vi "Kalibrierung laden.vi"() -> ()   [LabVIEW 2020, in "FT-IR.lvlib" / "Spanfaktor.lvlib"]
uses:
  Spanfaktor.lvlib
  FGV FT-IR Aktionen.ctl
  Sprachverwaltung/FGV Aktion Tabelle zerlegen.ctl
  FGV FT-IR Gasliste Aktionen.ctl
  Aktion FGV Span.ctl
  Aktionen EVID-Codes.ctl
  FT-IR.lvlib
  Allgemein/allgemeine Sub-VIs.lvlib
  TOOLweb Interface Library/TOOLweb Interface.lvlib
  Sprachverwaltung/Sprachverwaltung.lvlib
panel:
  out "Offset alt":string
  out "Offset neu":string
  out "Spanfaktor alt":string
  out "Spanfaktor Neu":string caption="Spanfaktor neu"
  out "Kalibrierung für Komponente":string
  # "Kalibrierdaten laden"
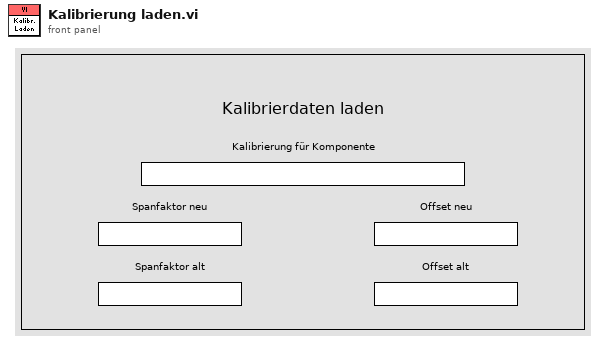
[diagram p1: front panel]
types:
  T1 = typedef "Sprachverwaltung.lvlib/FGV Aktion Tabelle zerlegen.ctl" = enum16{"laden", "vereinzeln", "speichern"}
  T2 = typedef "FT-IR.lvlib/FGV FT-IR Aktionen.ctl" = enum16{"lesen", "NOG setzen", "NOS setzen", "Initialisieren", "speichern", "ALLES setzen", "FT-IR Spektrum loggen", "Komm Stoppen", "Spektrum LogKonfig"}
  T3 = typedef "FT-IR.lvlib/Aktionen EVID-Codes.ctl" = enum16{"lesen", "setzen", "laden", "speichern", "1Hz/5Hz", "Smoothing", "Rolling Average"}
  T4 = typedef "FT-IR.lvlib/FGV FT-IR Gasliste Aktionen.ctl" = enum16{"lesen", "Gasliste FT-IR", "Gasliste ausgelesen", "laden", "speichern", "löschen"}
  T5 = typedef "FT-IR.lvlib/Spanfaktor.lvlib/Aktion FGV Span.ctl" = enum16{"lesen", "Span", "Seite aktiv", "Offset", "FGV aktualisiert", "Aktualisierung aufheben"}
  T6 = typedef "String - Ausgabefeld.ctl" = string
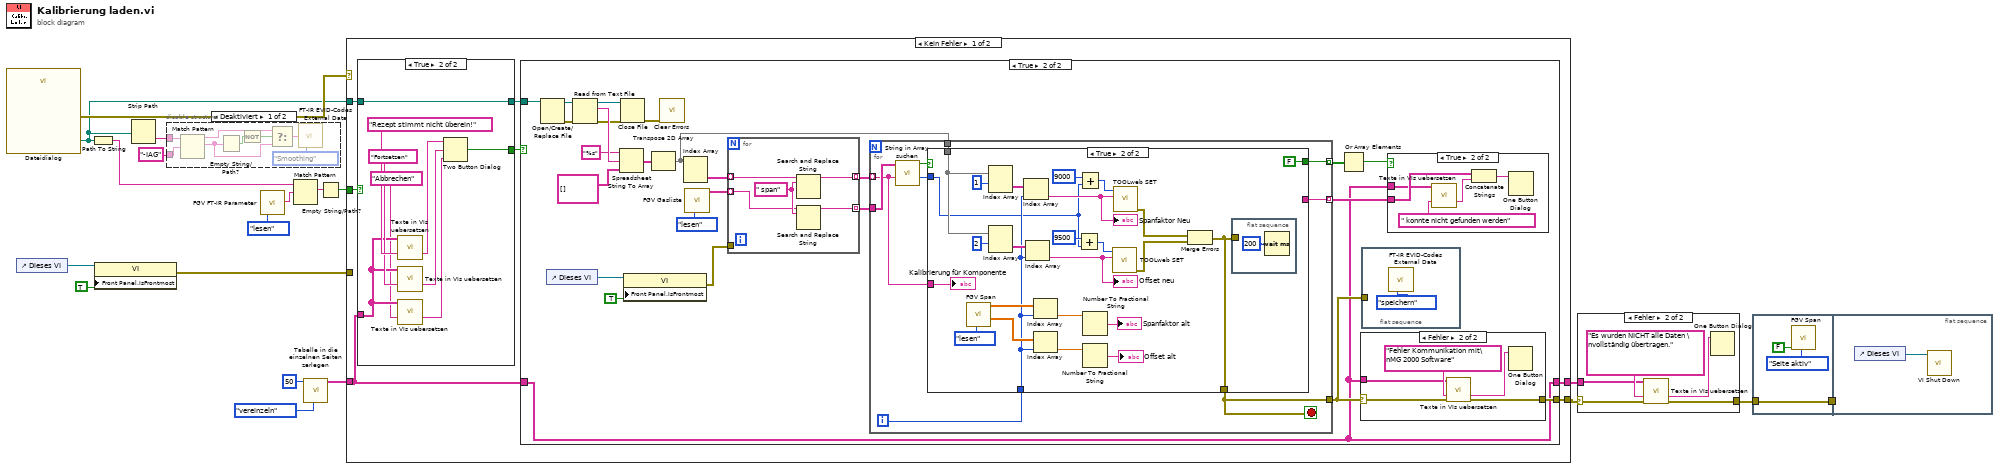
[diagram p0: block diagram]
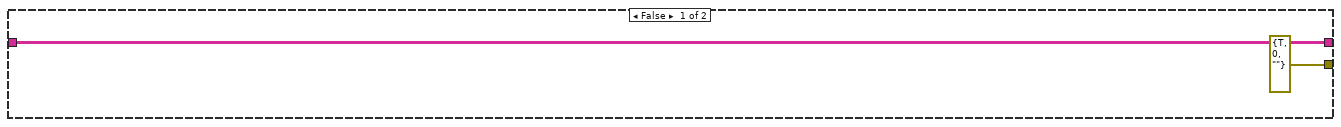
[diagram p3: hidden frame]
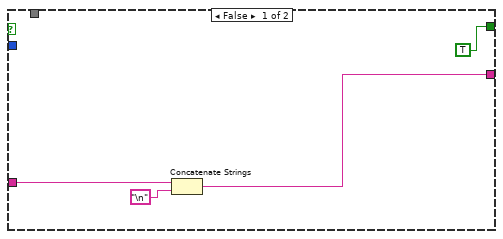
[diagram p6: hidden frame]
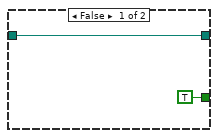
[diagram p7: hidden frame]
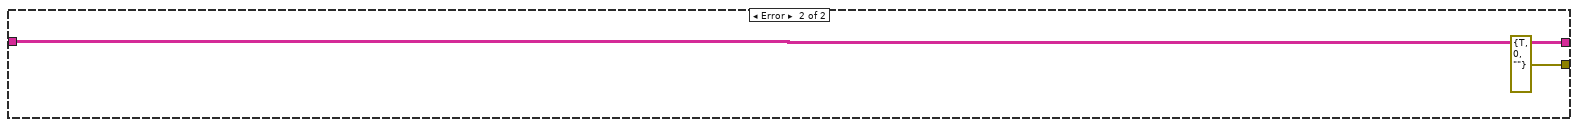
[diagram p8: hidden frame]
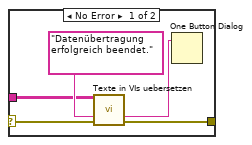
[diagram p9: hidden frame]
diagram:
  n1 = call "Dateidialog"() -> ("selected path"=w9:path, "error out"=w12:errorcluster)  [unwired: 12 in, 2 out]
  n2 = control-ref of="Dieses VI"() -> (w7:refnum<vi>)
  n3 = Path To String(path=w9) -> (string=w10:string)
  n4 = property class="VI"(reference=w7, "Front Panel.IsFrontmost"=TRUE ("Frontpanel-Fenster:Ist im Vordergrund")) -> (error out=w5:errorcluster)  [unwired: 1 in, 1 out]
  n5 = Strip Path(path=w9) -> (name=w8:string)  [unwired: 1 out]
  n6 = disable-structure shown="Deaktiviert" {
    disable-tunnel: "-IAG" ("Regulärer Ausdruck") -> [w27 _]
    disable-tunnel: w8 -> [w25 _]
    frame Disabled {
      n7 = Match Pattern(string=w25, regular expression=w27) -> (before substring=w22:string, match substring=w21:string)  [unwired: 1 in, 2 out]
      n8 = Empty String/Path?(string/path=w21) -> (empty?=w24:bool)
      n9 = Not(x=w24) -> (.not. x?=w20:bool)
      n10 = Select(t=w22, s=w20, f=w21) -> (s? t:f=w23:string)
      n11 = call "FT-IR EVID-Codes External Data.vi"("Rolling Average Settings"=w23, "Aktionen"=Aktionen_EVID-Codes."Smoothing") -> ()  [unwired: 8 in, 6 out]
    }
    frame Enabled {
    }
  }
  n12 = call "FGV FT-IR Parameter.vi"("Aktion"=FGV_FT-IR_Aktionen."lesen") -> ("Current Recipe"=w18:string)  [unwired: 11 in, 7 out]
  n13 = Match Pattern(string=w10, regular expression=w18) -> (match substring=w17:string)  [unwired: 1 in, 3 out]
  n14 = call "Tabelle in die einzelnen Seiten zerlegen.vi"("Aktion"=FGV_Aktion_Tabelle_zerlegen."vereinzeln", "Index (Seite)"=50) -> ("Sprachliste"=w2:string[][])  [unwired: 7 in, 2 out]
  n15 = Empty String/Path?(string/path=w17) -> (empty?=w16:bool)
  n16 = case shown="Kein Fehler" w12 {
    tunnel: w16 -> [w34 _]
    tunnel: w9 -> [w33 _]
    tunnel: [w30 errorcluster {"status"=TRUE, "code"=0, "source"=""} ("error IO")] -> w15
    tunnel: w5 -> [_ _]
    tunnel: w2 -> [w29 w129]
    tunnel: [w28 w129] -> w1
    frame No Error {
      n17 = case shown="True" w34 {
        tunnel: w33 -> [w119 w127]
        tunnel: [TRUE ("T button?") w128] -> w32
        tunnel: [w119 w127] -> w31
        tunnel: w29 -> [_ w122]
        frame False {
        }
        frame True {
          n18 = call "Texte in VIs uebersetzen.vi"("Sprachliste"=w122, "String zum Übersetzen"="Rezept stimmt nicht überein!" ("Nachricht")) -> ("String zum Übersetzen"=w125:string)  [unwired: 9 in, 4 out]
          n19 = call "Texte in VIs uebersetzen.vi"("Sprachliste"=w122, "String zum Übersetzen"="Fortsetzen" ("Text für T-Schaltfläche (\"OK\")")) -> ("String zum Übersetzen"=w123:string)  [unwired: 9 in, 4 out]
          n20 = call "Texte in VIs uebersetzen.vi"("Sprachliste"=w122, "String zum Übersetzen"="Abbrechen" ("Text für F-Schaltfläche (\"Abbrechen\")")) -> ("String zum Übersetzen"=w120:string)  [unwired: 9 in, 4 out]
          n21 = Two Button Dialog(message=w125, 1:w120, 2:w123) -> (T button?=w128:bool)
        }
      }
      n22 = case shown="True" w32 {
        tunnel: w31 -> [_ w52]
        tunnel: [errorcluster {"status"=TRUE, "code"=0, "source"=""} ("error IO") w45] -> w30
        tunnel: w29 -> [w35 w37]
        tunnel: [w35 w37] -> w28
        frame False {
        }
        frame True {
          n23 = Open/Create/Replace File(file path (use dialog)=w52) -> (refnum out=w61:refnum<file>, error out=w53:errorcluster)  [unwired: 1 in, 5 out]
          n24 = control-ref of="Dieses VI"() -> (w39:refnum<vi>)
          n25 = Read from Text File(file (use dialog)=w61, error in=w53) -> (refnum out=w60:refnum<file>, text=w59:string, error out=w56:errorcluster)  [unwired: 3 out]
          n26 = Spreadsheet String To Array(format string="%s" ("Format-String"), spreadsheet string=w59, array type (2D Dbl)=string[][] []) -> (array=w58:string[][])  [unwired: 1 out]
          n27 = Close File(refnum=w60, error in=w56) -> (error out=w57:errorcluster)  [unwired: 1 out]
          n28 = property class="VI"(reference=w39, "Front Panel.IsFrontmost"=TRUE ("Frontpanel-Fenster:Ist im Vordergrund")) -> (error out=w38:errorcluster)  [unwired: 1 in, 1 out]
          n29 = Transpose 2D Array(2D array=w58) -> (transposed array=w46:string[][])
          n30 = call <vilib>:"Clear Errors.vi"("error in (no error)"=w57) -> ()  [unwired: 5 in, 2 out]
          n31 = Index Array(array=w46) -> (element=w50:string[])  [unwired: 2 in]
          n32 = call "FGV Gasliste.vi"("Aktionen"=FGV_FT-IR_Gasliste_Aktionen."lesen") -> ("Aktuelle Gasliste FT-IR"=w49:T6[])  [unwired: 8 in, 2 out]
          n33 = for {
            tunnel: w50 -> [w114] mode=indexing
            tunnel: w49 -> [w113] mode=indexing
            tunnel: [w116] -> w48 mode=indexing
            tunnel: [w115] -> w47 mode=indexing
            tunnel: w38 -> [_]
            w117 = " span"
            n34 = Search and Replace String(input string=w114, search string=w117) -> (result string=w116:string)  [unwired: 6 in, 3 out]
            n35 = Search and Replace String(input string=w113, search string=w117) -> (result string=w115:string)  [unwired: 6 in, 3 out]
          }
          n36 = for {
            tunnel: w48 -> [w78] mode=indexing
            tunnel: w47 -> [w82]
            tunnel: w46 -> [w80]
            tunnel: [w77] -> w44
            tunnel: [w75] -> w41 mode=indexing
            tunnel: [w74] -> w43 mode=indexing
            i -> [w76]
            stop <- w77 stop-if-true
            n37 = call "String in Array suchen.vi"("Nach String/Zeichen suchen (-)"=w78, "String-Array"=w82) -> ("Index"=w79:i32, "Gefunden?"=w81:bool)  [unwired: 7 in, 1 out]
            n38 = case shown="True" w81 {
              tunnel: w80 -> [_ w111]
              tunnel: w79 -> [_ w88]
              tunnel: w78 -> [w86 w108]
              tunnel: [_ w92] -> w77
              tunnel: w76 -> [_ w89]
              tunnel: [w84 _] -> w75
              tunnel: [TRUE FALSE] -> w74
              frame False {
                n39 = Concatenate Strings(w86, "\n") -> (w84:string)
              }
              frame True {
                n40 = call "FGV Span.vi"("Aktion"=Aktion_FGV_Span."lesen") -> ("Offset"=w99:sgl[], "Span"=w100:sgl[])  [unwired: 7 in, 2 out]
                n41 = Index Array(array=w111, index (row)=1 ("Index (Zeile)")) -> (element=w110:string[])  [unwired: 1 in]
                n42 = Index Array(array=w111, index (row)=2 ("Index (Zeile)")) -> (element=w109:string[])  [unwired: 1 in]
                n43 = Index Array(array=w110, index=w89) -> (element=w103:string)
                "Spanfaktor Neu" <- w103
                n44 = Index Array(array=w109, index=w89) -> (element=w102:string)
                "Offset neu" <- w102
                n45 = Index Array(array=w100, index=w89) -> (element=w98:sgl)
                n46 = Index Array(array=w99, index=w89) -> (element=w97:sgl)
                n47 = Add(x=9500, y=w88) -> (x+y=w105:i32)
                n48 = Add(x=9000, y=w88) -> (x+y=w106:i32)
                n49 = Number To Fractional String(number=w98) -> (F-format string=→"Spanfaktor alt":string)  [unwired: 3 in]
                n50 = Number To Fractional String(number=w97) -> (F-format string=→"Offset alt":string)  [unwired: 3 in]
                n51 = call "TOOLweb SET.vi"("Wert-String"=w102, "EVID-Nummer"=w105) -> ("error out"=w93:errorcluster)  [unwired: 3 in, 2 out]
                n52 = call "TOOLweb SET.vi"("Wert-String"=w103, "EVID-Nummer"=w106) -> ("error out"=w94:errorcluster)  [unwired: 3 in, 2 out]
                n53 = Merge Errors(w94, w93) -> (w92:errorcluster)
                n54 = flat-sequence {
                  tunnel: w92 -> [_]
                  frame #0 {
                    n55 = Wait (ms)(milliseconds to wait=u32 200 ("Zu wartende ms")) -> ()  [unwired: 1 out]
                  }
                }
                "Kalibrierung für Komponente" <- w108
              }
            }
          }
          n56 = Or Array Elements(Boolean array=w43) -> (logical OR=w42:bool)
          n57 = case shown="Fehler" w44 {
            selector: w44 -> [w68 w70]
            tunnel: [w68 w69] -> w45
            tunnel: w37 -> [_ w71]
            frame No Error {
            }
            frame Error {
              n58 = call "Texte in VIs uebersetzen.vi"("Sprachliste"=w71, "String zum Übersetzen"="Fehler Kommunikation mit\nMG 2000 Software" ("String"), "error in (no error)"=w70) -> ("String zum Übersetzen"=w73:string, "error out"=w69:errorcluster)  [unwired: 8 in, 3 out]
              n59 = One Button Dialog(message=w73) -> ()  [unwired: 1 in, 1 out]
            }
          }
          n60 = flat-sequence {
            tunnel: w44 -> [_]
            frame #0 {
              n61 = call "FT-IR EVID-Codes External Data.vi"("Aktionen"=Aktionen_EVID-Codes."speichern") -> ()  [unwired: 9 in, 6 out]
            }
          }
          n62 = case shown="True" w42 {
            tunnel: w41 -> [_ w65]
            tunnel: w37 -> [_ w62]
            frame False {
            }
            frame True {
              n63 = call "Texte in VIs uebersetzen.vi"("Sprachliste"=w62, "String zum Übersetzen"=" konnte nicht gefunden werden" ("String")) -> ("String zum Übersetzen"=w63:string)  [unwired: 9 in, 4 out]
              n64 = Concatenate Strings(w65, w63) -> (w66:string)
              n65 = One Button Dialog(message=w66) -> ()  [unwired: 1 in, 1 out]
            }
          }
        }
      }
    }
    frame Error {
    }
  }
  n66 = case shown="Fehler" w15 {
    selector: w15 -> [w134 w138]
    tunnel: [w134 w137] -> w14
    tunnel: w1 -> [w131 w136]
    frame No Error {
      n67 = call "Texte in VIs uebersetzen.vi"("Sprachliste"=w131, "String zum Übersetzen"="Datenübertragung erfolgreich beendet." ("String")) -> ("String zum Übersetzen"=w132:string)  [unwired: 9 in, 4 out]
      n68 = One Button Dialog(message=w132) -> ()  [unwired: 1 in, 1 out]
    }
    frame Error {
      n69 = call "Texte in VIs uebersetzen.vi"("Sprachliste"=w136, "String zum Übersetzen"="Es wurden NICHT alle Daten \nvollständig übertragen." ("String"), "error in (no error)"=w138) -> ("String zum Übersetzen"=w135:string, "error out"=w137:errorcluster)  [unwired: 8 in, 3 out]
      n70 = One Button Dialog(message=w135) -> ()  [unwired: 1 in, 1 out]
    }
  }
  n71 = flat-sequence {
    tunnel: w14 -> [w142]
    tunnel: [w142] -> w13
    tunnel: w13 -> [_]
    frame #0 {
      n72 = call "FGV Span.vi"("Aktion"=Aktion_FGV_Span."Seite aktiv", "Aktiv"=FALSE) -> ()  [unwired: 6 in, 4 out]
    }
    frame #1 {
      n73 = control-ref of="Dieses VI"() -> (w143:refnum<vi>)
      n74 = call "VI Shut Down.vi"("VI Referenz"=w143) -> ()  [unwired: 11 in]
    }
  }
